vi "Stop.vi"(8 "error in (no error)":errorcluster, 10 "Message in":refnum<class "StopMessage.lvclass">, 11 "ImageStack in":refnum<class "ImageStack.lvclass">) -> (0 "error out":errorcluster, 3 "ImageStack out":refnum<class "ImageStack.lvclass">)   [LabVIEW 2012, in "ImageStack.lvclass"]
doc: "This member function is called when the statemachine in the run.vi receives an 'stop' command. It relays the message to all observers of the component.\n\nOverride this member function in your derived class if you need additional stop functionality (but don't forget to call the parent method)."
uses:
  ImageStack.lvclass
  <vilib>/Distrio/Murmex/StopMessage/StopMessage.lvclass
  <vilib>/Distrio/Murmex/Murmex/Murmex.lvclass
  ImageStack.lvclass/ImageStack.ctl
  <vilib>/Distrio/Murmex/GenericMessage/GenericMessage.lvclass
  <vilib>/Distrio/Murmex/Message/Add or replace parameter.vi
  <vilib>/Distrio/Murmex/Message/Message.lvclass
panel:
  # "This method is called when the STOP\ntrigger is sent. \n\nOverride this method when your component needs to\nrespond to this trigger. \n\nCall parent for proper implementation"
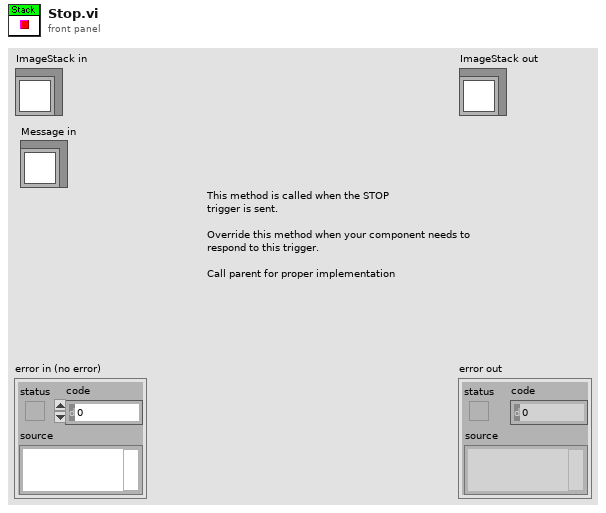
[diagram p1: front panel]
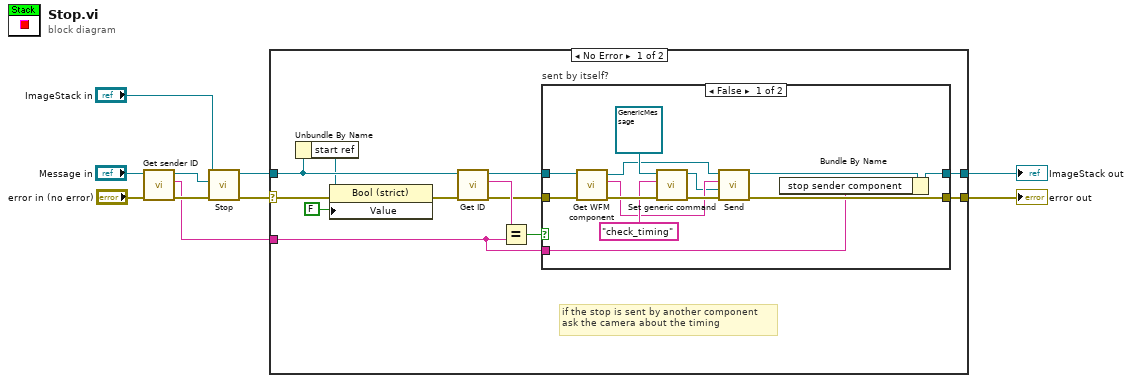
[diagram p0: block diagram]
diagram:
  n1 = call <vilib>:"Get sender ID.vi"("error in (no error)"="error in (no error)", "Message in"="Message in") -> ("error out"=w6:errorcluster, "sender"=w3:string, "Message out"=w4:refnum<class "StopMessage.lvclass">)  [unwired: 7 in]
  n2 = call-parent "Stop.vi"("error in (no error)"=w6, "Message in"=w4, "Murmex in"="ImageStack in") -> ("error out"=w1:errorcluster, "Murmex out"=w2:refnum<class "ImageStack.lvclass">)  [unwired: 7 in]
  n3 = case shown="No Error" w1 {
    selector: w1 -> [w21 w39]
    tunnel: [w17 w39] -> w8
    tunnel: [w18 w38] -> w9
    tunnel: w3 -> [w16 _]
    tunnel: w2 -> [w15 w38]
    frame No Error {
      # "if the stop is sent by another component\nask the camera about the timing"
      n4 = Unbundle By Name(w15) -> ("start ref"=w14:refnum<vi>)
      n5 = property class="Bool (strict)"(reference=w14, error in=w21, "Value"=FALSE) -> (error out=w20:errorcluster)  [unwired: 1 out]
      n6 = call <vilib>:"Get ID.vi"("error in (no error)"=w20, "Murmex in"=w15) -> ("error out"=w12:errorcluster, "component id"=w19:string, "Murmex out"=w13:refnum<class "ImageStack.lvclass">)  [unwired: 7 in]
      n7 = Equal?(x=w19, y=w16) -> (x = y?=w11:bool)
      n8 = case "sent by itself?" shown="False" w11 {
        tunnel: [w24 w37] -> w18
        tunnel: w13 -> [w35 w37]
        tunnel: [w29 w36] -> w17
        tunnel: w12 -> [w34 w36]
        tunnel: w16 -> [w23 _]
        frame False {
          n9 = call-dynamic "Get WFM component.vi"("error in (no error)"=w34, "ImageStack in"=w35) -> ("error out"=w33:errorcluster, "Wavefront component name"=w28:string, "ImageStack out"=w27:refnum<class "ImageStack.lvclass">)  [unwired: 7 in]
          n10 = call <vilib>:"Set generic command.vi"("error in (no error)"=w33, "generic command"="check_timing", "GenericMessage in"=refnum<class "GenericMessage.lvclass"> refnum ("Distrio Murmex 1.2:GenericMessage")) -> ("error out"=w30:errorcluster, "GenericMessage out"=w26:refnum<class "GenericMessage.lvclass">)  [unwired: 7 in]
          n11 = call <vilib>:"Send.vi"("error in (no error)"=w30, "Message"=w26, "recipient"=w28, "Murmex in"=w27) -> ("error out"=w29:errorcluster, "Murmex out"=w25:refnum<class "ImageStack.lvclass">)  [unwired: 6 in]
          n12 = Bundle By Name(cluster=w25, "stop sender component"=w23) -> (w24:refnum<class "ImageStack.lvclass">)
        }
        frame True {
        }
      }
    }
    frame Error {
    }
  }
  "error out" <- w8
  "ImageStack out" <- w9
